vi "Shooter_Fire_1_20.vi"(8 "CamPos":dbl, 9 "PotPos In":dbl, 10 "FireButton":bool, 11 "IsReady":bool) -> (0 "CamPow":dbl, 1 "CamPosOut":dbl, 3 "PotPosOut":dbl)   [LabVIEW 2013]
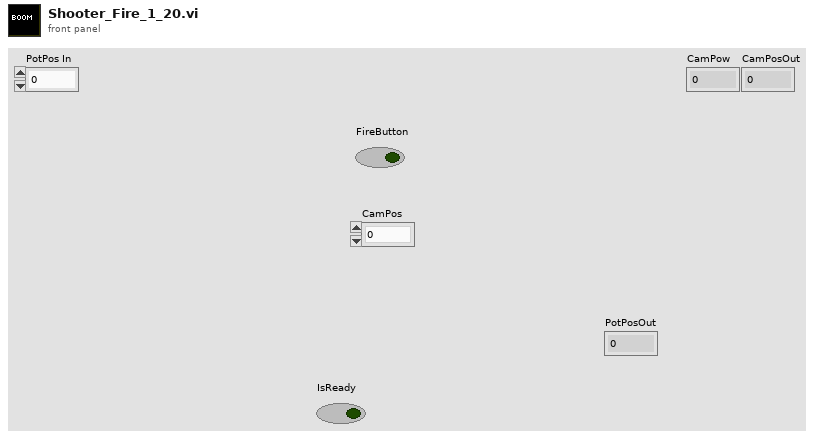
[diagram p1: front panel]
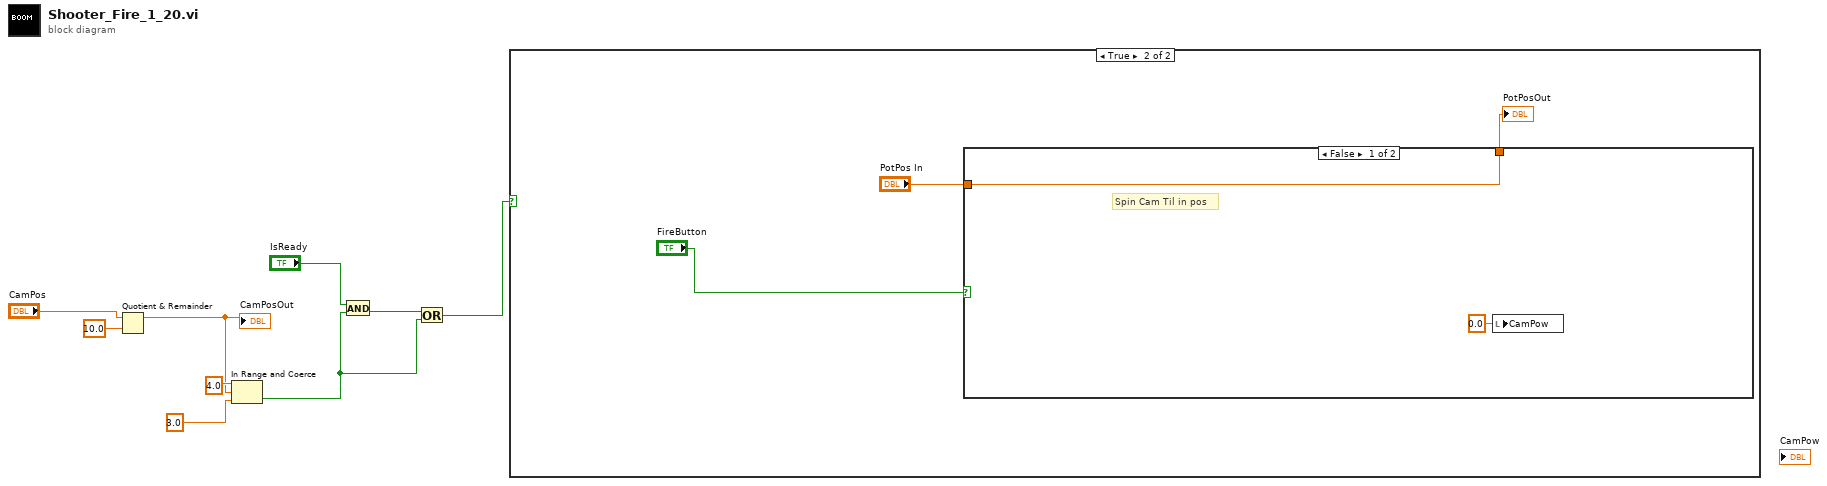
[diagram p0: block diagram]
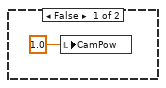
[diagram p2: hidden frame]
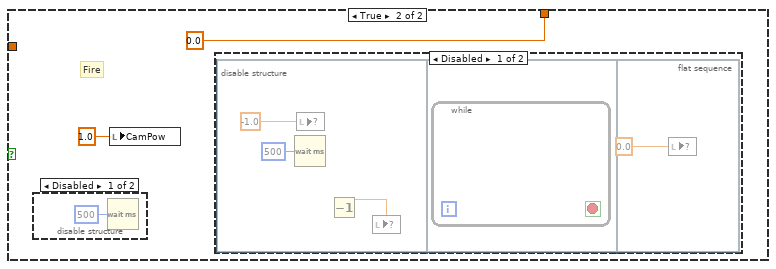
[diagram p3: hidden frame]
diagram:
  n1 = Quotient & Remainder(x="CamPos", y=10.0) -> (x-y*floor(x/y)=w2:dbl)  [unwired: 1 out]
  "CamPosOut" <- w2
  n2 = In Range and Coerce(upper limit=4.0 ("x"), x=w2, lower limit=3.0 ("y")) -> (In Range?=w4:bool)  [unwired: 1 out]
  n3 = And(x="IsReady", y=w4) -> (x .and. y?=w6:bool)
  n4 = Or(x=w6, y=w4) -> (x .or. y?=w5:bool)
  n5 = case shown="True" w5 {
    frame False {
      n6 = local write "CamPow"(1.0 ("CamPower")) -> ()
    }
    frame True {
      n7 = case shown="False" "FireButton" {
        tunnel: [w14 0.0] -> w12
        tunnel: "PotPos In" -> [w14 _]
        frame False {
          # "Spin Cam Til in pos"
          n8 = local write "CamPow"(0.0 ("CamPos")) -> ()
        }
        frame True {
          # "Fire"
          n9 = disable-structure shown="Disabled" {
            frame Disabled {
              n10 = Wait (ms)(milliseconds to wait=u32 500) -> ()  [unwired: 1 out]
            }
            frame Enabled {
            }
          }
          n11 = local write "CamPow"(1.0 ("CamPower")) -> ()
          n12 = disable-structure shown="Disabled" {
            frame Disabled {
              n13 = flat-sequence {
                frame #0 {
                  n14 = Wait (ms)(milliseconds to wait=u32 500) -> ()  [unwired: 1 out]
                  n15 = local write item#-1(-1.0 ("CamPower")) -> ()
                  n16 = Decrement() -> (x-1=w19:dbl)  [unwired: 1 in]
                  n17 = local write item#-1(w19) -> ()
                }
                frame #1 {
                  n18 = while {
                    stop <- _ stop-if-true
                  }
                }
                frame #2 {
                  n19 = local write item#-1(0.0 ("CamPower")) -> ()
                }
              }
            }
            frame Enabled {
            }
          }
        }
      }
      "PotPosOut" <- w12
    }
  }
